vi "Write FunctionCreateFileHandler.vi"(8 "error in (no error)":errorcluster, 10 "FunctionCreateFileHandler":string="create_file_handler", 11 "Logger in":refnum<class "Logger.lvclass">) -> (0 "error out":errorcluster, 3 "Logger out":refnum<class "Logger.lvclass">)   [LabVIEW 2022 SP3, in "Logger.lvlib" / "Logger.lvclass"]
uses:
  Logger.lvclass
  Logger.lvclass/Logger.ctl
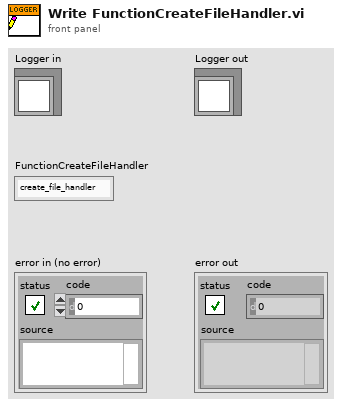
[diagram p1: front panel]
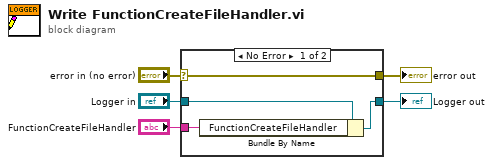
[diagram p0: block diagram]
diagram:
  n1 = case shown="No Error" "error in (no error)" {
    selector: "error in (no error)" -> [w9 w10]
    tunnel: [w9 w10] -> w4
    tunnel: [w7 w11] -> w2
    tunnel: "Logger in" -> [w8 w11]
    tunnel: "FunctionCreateFileHandler" -> [w6 _]
    frame No Error {
      n2 = Bundle By Name(cluster=w8, "FunctionCreateFileHandler"=w6) -> (w7:refnum<class "Logger.lvclass">)
    }
    frame Error {
    }
  }
  "error out" <- w4
  "Logger out" <- w2
